vi "Keithley617_Read_GPIB.vi"(7 "GPIB Address String":string="27", 8 "Error In":errorcluster) -> (0 "Error Out":errorcluster, 3 "Output value":dbl)   [LabVIEW 2015, in "Keithley617.lvlib"]
uses:
  Keithley617.lvlib
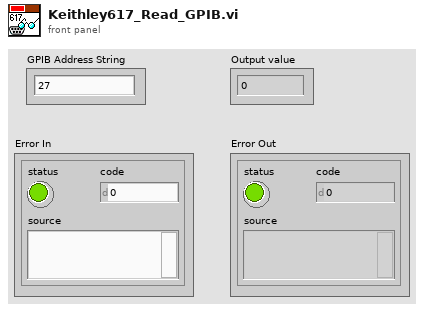
[diagram p1: front panel]
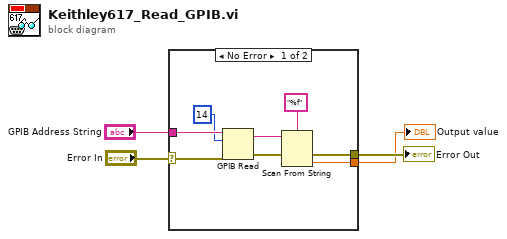
[diagram p0: block diagram]
diagram:
  n1 = case shown="No Error" "Error In" {
    selector: "Error In" -> [w10 w13]
    tunnel: "GPIB Address String" -> [w12 _]
    tunnel: [w6 w13] -> w2
    tunnel: [w5 _] -> w1
    frame No Error {
      n2 = GPIB Read(0:w12, 1:14 ("byte count"), 3:w10) -> (5:w9:string, 7:w8:errorcluster)  [unwired: 2 in, 1 out]
      n3 = Scan From String(format string="%f", input string=w9, error in=w8) -> (error out=w6:errorcluster, output 1=w5:dbl)  [unwired: 2 in, 2 out]
    }
    frame Error {
    }
  }
  "Error Out" <- w2
  "Output value" <- w1
